vi "Configure Output Synchronization.vi"(8 "error in (no error)":errorcluster, 9 "Output Synchronization Type (4: Waveform Synchronization)":u16(ring)=4 items=["Trigger", "Sweep Synchronization", "Phase-Locking", "Position Marker", "Waveform Synchronization", "Phase Zero", "Burst Done", "Sequence Synchronization"], 10 "Output Synchronization Operation (0: Auto)":u16(ring) items=["Auto ", "Manual ", "Off"], 11 "VISA resource name":refnum<visa-resource-name>) -> (0 "error out":errorcluster, 3 "VISA resource name out":refnum<visa-resource-name>)   [LabVIEW 2015, in "Fluke 28x Series.lvlib"]
doc: "Configures an output that is synchronized to some property of the carrier wave output, like the end of the waveform or the sweep frequency. This property can be automatically or manually controlled by the types specified in <b>Output Synchronization Type</b>."
uses:
  <instrlib>/Fluke 28x Series/Fluke 28x Series.lvlib
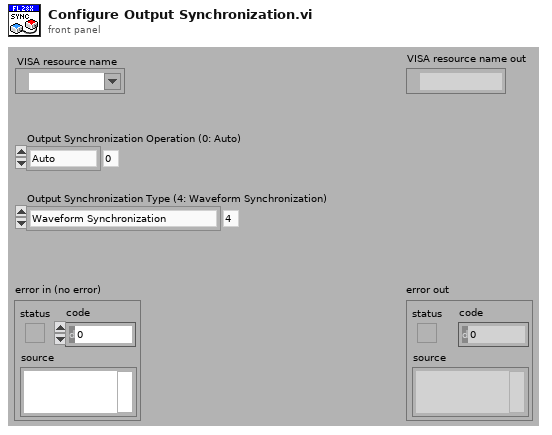
[diagram p1: front panel]
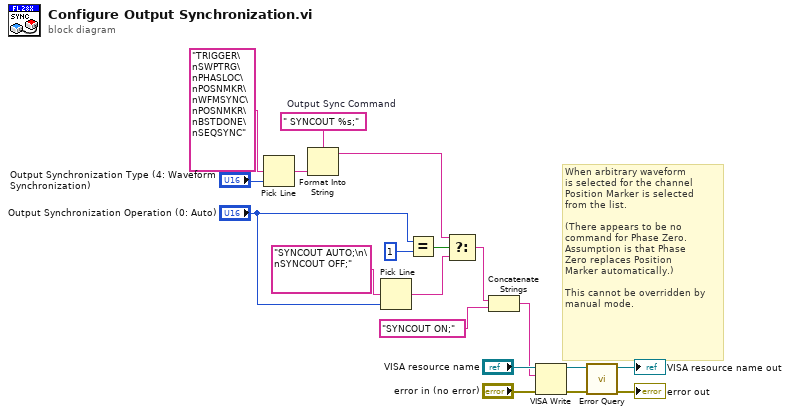
[diagram p0: block diagram]
diagram:
  w10 = " SYNCOUT %s;"  # Output Sync Command
  # "When arbitrary waveform\nis selected for the channel\nPosition Marker is selected\nfrom the list.\n \n(There appears to be no \ncommand for Phase Zero. \nAssumption is that Phase\nZero replaces Position \nMarker automatically.) \n\nThis cannot be overridden by \nmanual mode."
  n1 = Pick Line(multi-line string="TRIGGER\nSWPTRG\nPHASLOC\nPOSNMKR\nWFMSYNC\nPOSNMKR\nBSTDONE\nSEQSYNC", line index="Output Synchronization Type (4: Waveform Synchronization)") -> (output string=w11:string)  [unwired: 1 in]
  n2 = Format Into String(format string=w10, w11) -> (resulting string=w9:string)  [unwired: 2 in, 1 out]
  n3 = Pick Line(multi-line string="SYNCOUT AUTO;\n\nSYNCOUT OFF;", line index="Output Synchronization Operation (0: Auto)") -> (output string=w6:string)  [unwired: 1 in]
  n4 = Equal?(x="Output Synchronization Operation (0: Auto)", y=u16 1) -> (x = y?=w14:bool)
  n5 = Select(t=w9, s=w14, f=w6) -> (s? t:f=w3:string)
  n6 = Concatenate Strings(w3, "SYNCOUT ON;" ("string")) -> (w1:string)
  n7 = VISA Write(VISA resource name="VISA resource name", write buffer=w1, error in (no error)="error in (no error)") -> (VISA resource name out=w17:refnum<visa-resource-name>, error out=w18:errorcluster)  [unwired: 1 out]
  n8 = call <instrlib>:"Error Query.vi"("error in (no error)"=w18, "VISA resource name"=w17) -> ("error out"=→"error out":errorcluster, "VISA resource name out"=→"VISA resource name out":refnum<visa-resource-name>)  [unwired: 6 in, 2 out]
